vi "Serial_TCS_test.vi"() -> ()   [LabVIEW 2011]
uses:
  <vilib>/Instr/_visa.llb/VISA Configure Serial Port (Instr).vi
panel:
  out "DST?":bool
  out "error out":errorcluster
  out "Q String 2":string
  out "Q String":string
  out "Erreur?":bool
  in  "VISA resource name":refnum<visa-resource-name>="COM4"
  in  "baud rate (9600)":u32=57600
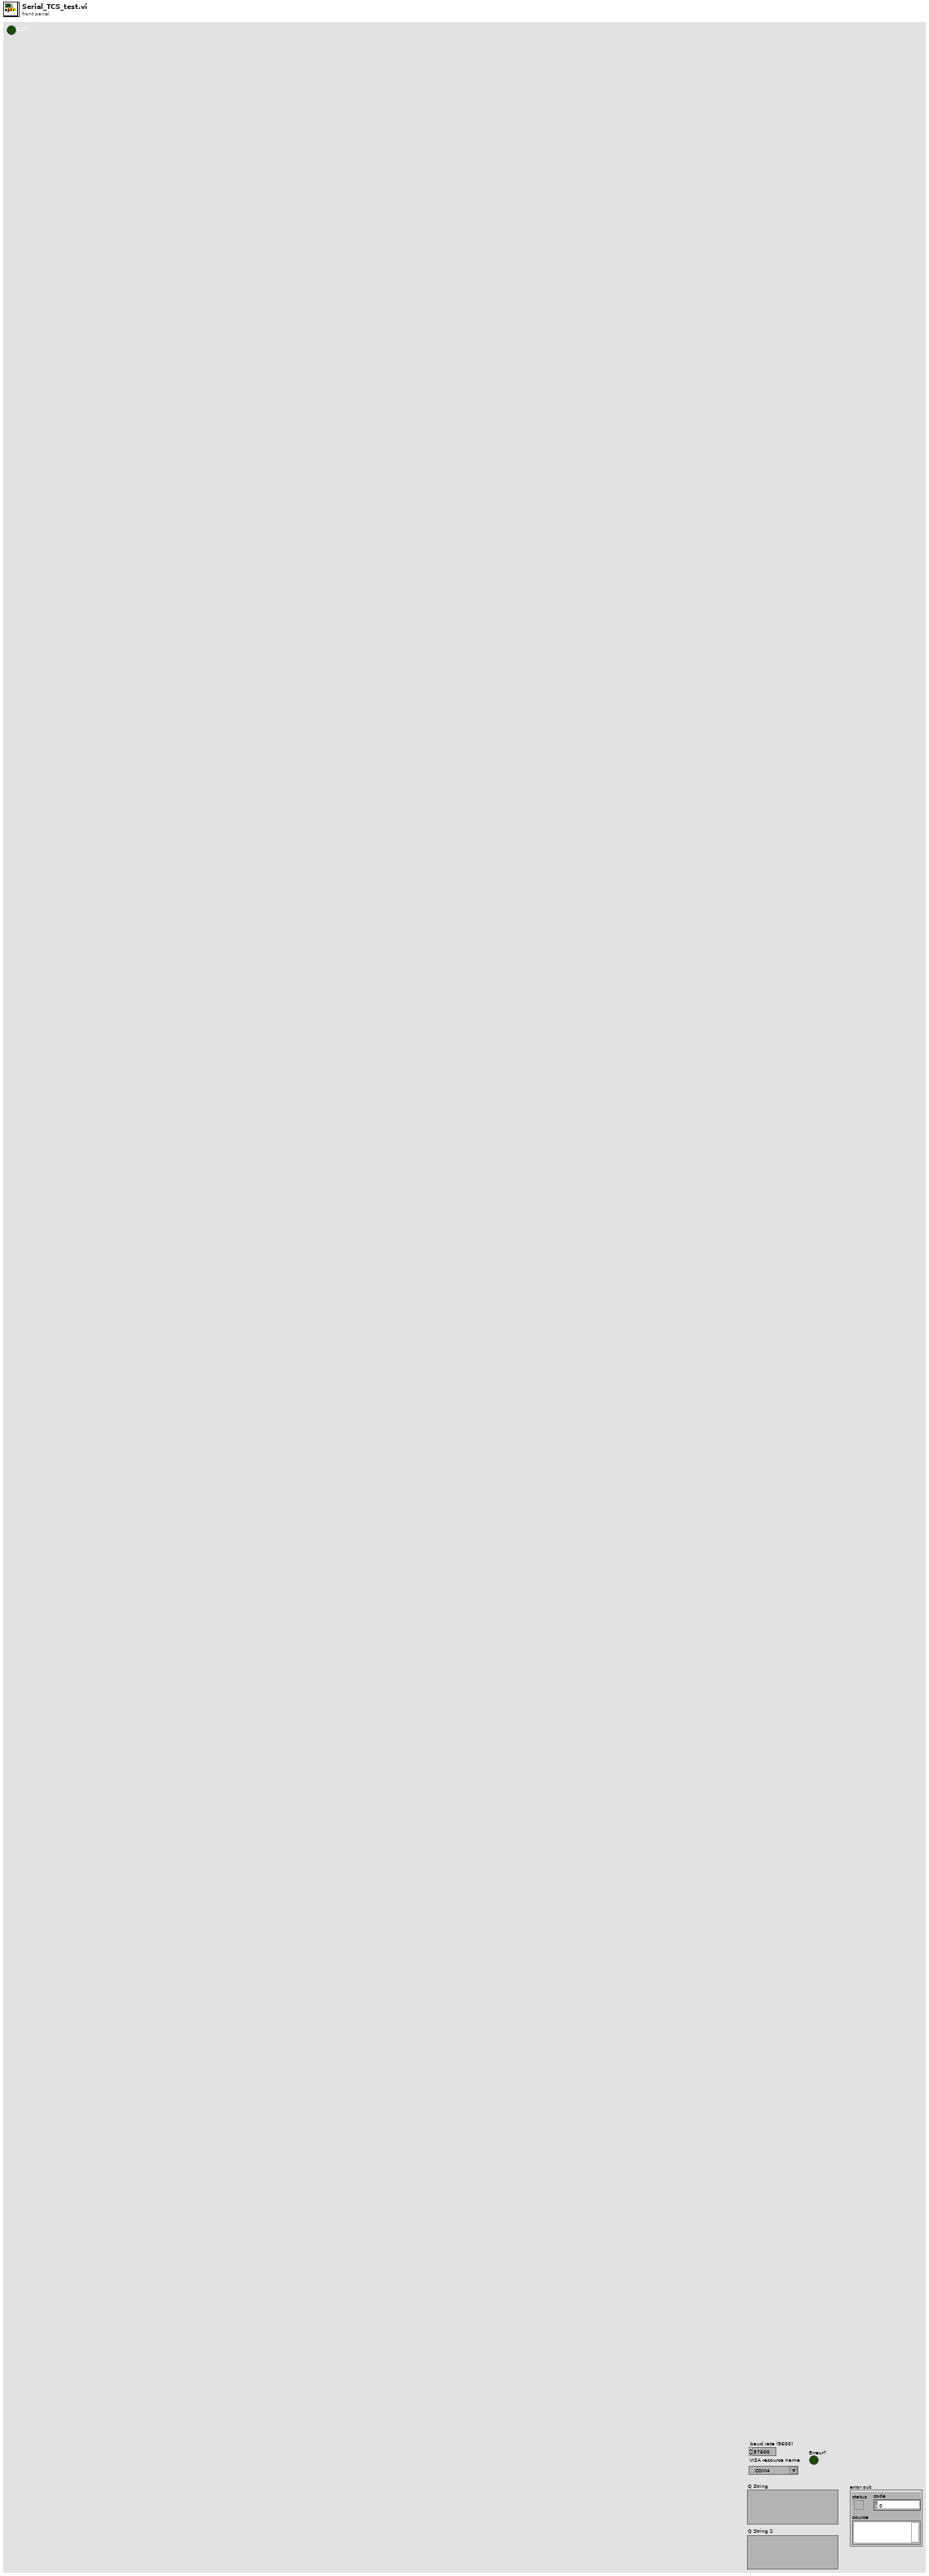
[diagram p1: front panel]
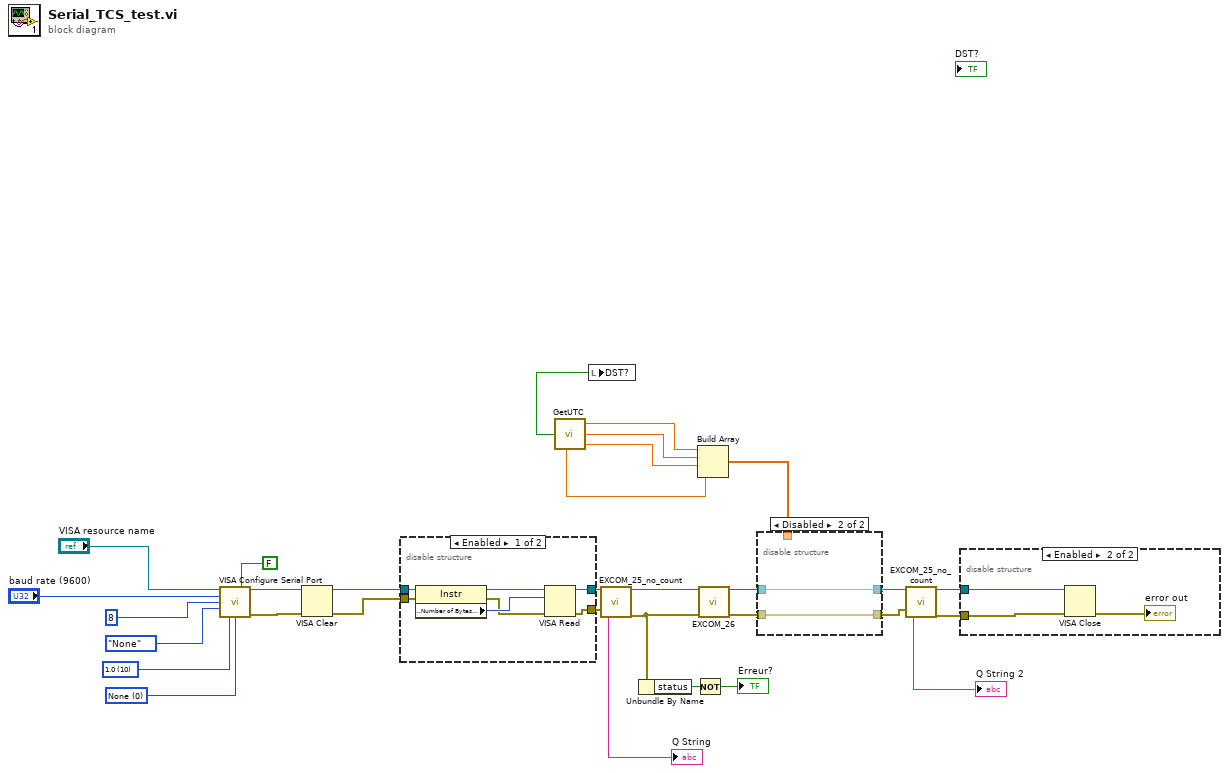
[diagram p0: block diagram]
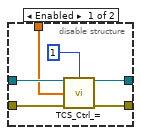
[diagram p2: hidden frame]
diagram:
  w30 = u16 0 items=["None", "XON/XOFF", "RTS/CTS", "XON/XOFF & RTS/CTS", "DTR/DSR", "XON/XOFF & DTR/DSR"] ("flow control (0:none)")
  w29 = u16 10 items=["1.0"=10, "1.5"=15, "2.0"=20] ("stop bits (10: 1 bit)")
  n1 = call-poly "VISA Configure Serial Port"("VISA resource name"="VISA resource name", "Enable Termination\nChar (T)"=FALSE ("Enable Termination\nChar (T)"), "baud rate (9600)"="baud rate (9600)", "data bits (8)"=u16 8, "parity (0:none)"=enum16{"None", "Odd", "Even", "Mark", "Space"}."None", "stop bits (10: 1 bit)"=w29, "flow control (0:none)"=w30) -> ("VISA resource name out"=w4:refnum<visa-resource-name>, "error out"=w3:errorcluster)  [unwired: 7 in]
  n2 = VISA Clear(VISA resource name=w4, error in (no error)=w3) -> (VISA resource name out=w1:refnum<visa-resource-name>, error out=w2:errorcluster)
  n3 = disable-structure shown="Enabled" {
    disable-tunnel: [w38 w39] -> w26
    disable-tunnel: [w35 w40] -> w24
    disable-tunnel: w2 -> [w33 w39]
    disable-tunnel: w1 -> [w32 w40]
    frame Enabled {
      n4 = property class="Instr"(reference=w32, error in=w33) -> (reference out=w37:refnum<visa-resource-name>, error out=w34:errorcluster, "Serial Settings:Number of Bytes at Serial Port"=w36:u32)
      n5 = VISA Read(VISA resource name=w37, byte count=w36, error in (no error)=w34) -> (VISA resource name out=w35:refnum<visa-resource-name>, error out=w38:errorcluster)  [unwired: 2 out]
    }
    frame Disabled {
    }
  }
  n6 = call "GetUTC.vi"() -> ("DST?"=w10:bool, "UTC_fractional"=w6:dbl, "Year"=w9:dbl, "Month"=w8:dbl, "Day"=w7:dbl)  [unwired: 3 out]
  n7 = local write "DST?"(w10) -> ()
  n8 = call "EXCOM_25_no_count.vi"("VISA resource name"=w24, "error in"=w26) -> ("Q String"=→"Q String":string, "VISA resource name dup"=w19:refnum<visa-resource-name>, "error out"=w18:errorcluster)  [unwired: 3 in, 12 out]
  n9 = Unbundle By Name(w18) -> ("status"=w25:bool)
  n10 = Not(x=w25) -> (.not. x?=→"Erreur?":bool)
  n11 = Build Array(w9, w8, w7, w6) -> (w5:dbl[])
  n12 = call "EXCOM_26.vi"("VRN IN"=w19, "Error IN"=w18) -> ("VRN OUT"=w14:refnum<visa-resource-name>, "Error OUT"=w11:errorcluster)  [unwired: 7 in, 5 out]
  n13 = disable-structure shown="Disabled" {
    disable-tunnel: w14 -> [w46 w48]
    disable-tunnel: [w45 w48] -> w13
    disable-tunnel: [w44 w47] -> w12
    disable-tunnel: w11 -> [w43 w47]
    disable-tunnel: w5 -> [w41 _]
    frame Enabled {
      n14 = call "TCS_Ctrl_=.vi"("VRN IN"=w46, "Commande #"=1, "Args"=w41, "Error IN"=w43) -> ("VRN OUT"=w45:refnum<visa-resource-name>, "Error OUT"=w44:errorcluster)  [unwired: 9 in, 1 out]
    }
    frame Disabled {
    }
  }
  n15 = call "EXCOM_25_no_count.vi"("VISA resource name"=w13, "error in"=w12) -> ("Q String"=→"Q String 2":string, "VISA resource name dup"=w17:refnum<visa-resource-name>, "error out"=w16:errorcluster)  [unwired: 3 in, 12 out]
  n16 = disable-structure shown="Enabled" {
    disable-tunnel: w17 -> [_ w51]
    disable-tunnel: w16 -> [_ w50]
    frame Disabled {
    }
    frame Enabled {
      n17 = VISA Close(VISA resource name=w51, error in (no error)=w50) -> (error out=→"error out":errorcluster)
    }
  }
